vi "Acquire Data.vi"(8 "error in (no error)":errorcluster, 11 "USB Camera in":refnum<class "USB Camera.lvclass">) -> (0 "error out":errorcluster, 3 "USB Camera out":refnum<class "USB Camera.lvclass">)   [LabVIEW 2020, in "USB Camera.lvclass"]
uses:
  USB Camera.lvclass
  C:/Users/jharw/Documents/1 Folder to Rule them All/UMD/Inflation-Apparatus/src/Hardware/Sensors/Cameras/Camera.lvclass
  C:/Users/jharw/Documents/1 Folder to Rule them All/UMD/Inflation-Apparatus/src/Hardware/General Hardware.lvclass
  <vilib>/vision/driver/IMAQdx.llb/IMAQdx Buffer Number Mode.ctl
  General Hardware.lvclass/General Hardware.ctl
  USB Camera.lvclass/USB Camera.ctl
  Camera.lvclass/Camera.ctl
  Camera.lvclass
  General Hardware.lvclass
  <vilib>/vision/driver/NI_Vision_Acquisition_Software.lvlib
  <vilib>/vision/NI_Vision_Development_Module.lvlib
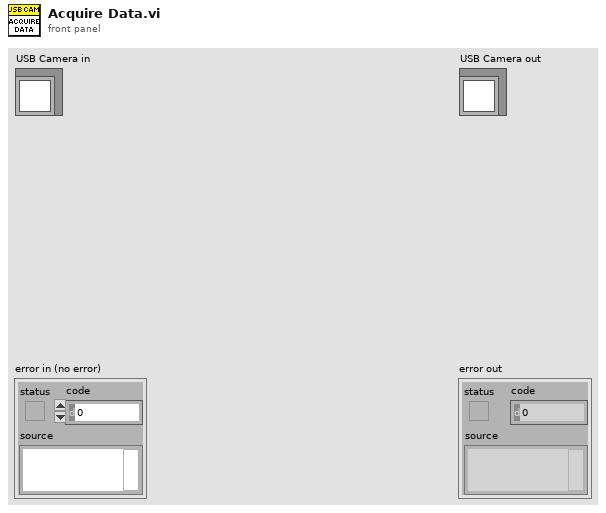
[diagram p1: front panel]
types:
  T1 = cluster{"Contrast":i32, "Filter width":i32, "Steepness":i32, "Subsampling Ratio":u32, "Show Search Area":bool, "Show Search Lines":bool, "Show Edges Found":bool, "Show Result":bool}
  T2 = typedef "NI_Vision_Acquisition_Software.lvlib/IMAQdx Buffer Number Mode.ctl" = enum32{"Next", "Last", "Buffer Number", "Every", "Last New"}
  T3 = typedef "IMAQdx.ctl" = refnum<k21>
  T4 = typedef "IMAQ Image.ctl" = refnum<image>
  T5 = typedef "IMAQ Rectangle" = cluster{"Left":i32, "Top":i32, "Right":i32, "Bottom":i32, "Rotation":dbl}
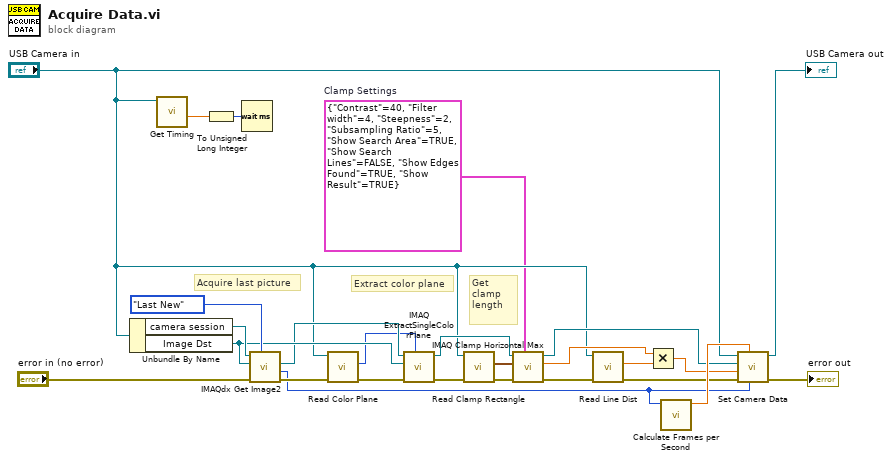
[diagram p0: block diagram]
diagram:
  w3 = T1 {"Contrast"=40, "Filter width"=4, "Steepness"=2, "Subsampling Ratio"=5, "Show Search Area"=TRUE, "Show Search Lines"=FALSE, "Show Edges Found"=TRUE, "Show Result"=TRUE}  # Clamp Settings
  # "Get clamp length"
  # "Extract color plane"
  # "Acquire last picture"
  n1 = Unbundle By Name("USB Camera in") -> ("camera session"=w20:T3, "Image Dst"=w16:T4)
  n2 = call "Get Timing.vi"("General Hardware in"="USB Camera in") -> ("time delay (ms)"=w22:dbl)  [unwired: 7 in, 3 out]
  n3 = To Unsigned Long Integer(number=w22) -> (unsigned 32bit integer=w23:u32)
  n4 = Wait (ms)(milliseconds to wait=w23) -> ()  [unwired: 1 out]
  n5 = call <vilib>:"IMAQdx Get Image2.vi"("Buffer Number Mode (Next)"=IMAQdx_Buffer_Number_Mode."Last New" ("Buffer Number Mode"), "error in"="error in (no error)", "Image In"=w16, "Session In"=w20) -> ("error out"=w18:errorcluster, "Buffer Number Out"=w2:u32, "Image Out"=w15:T4)  [unwired: 4 in, 1 out]
  n6 = call "Read Color Plane.vi"("error in (no error)"=w18, "Camera in"="USB Camera in") -> ("error out"=w17:errorcluster, "Color Plane"=w1:i32)  [unwired: 7 in, 1 out]
  n7 = call "IMAQ ExtractSingleColorPlane"("Color Plane"=w1, "error in (no error)"=w17, "Image Dst"=w16, "Image Src"=w15) -> ("error out"=w14:errorcluster, "Image Dst Out"=w11:T4)  [unwired: 6 in]
  n8 = call "Read Clamp Rectangle.vi"("error in (no error)"=w14, "Camera in"="USB Camera in") -> ("error out"=w13:errorcluster, "Rectangle"=w12:T5)  [unwired: 7 in, 1 out]
  n9 = call "IMAQ Clamp Horizontal Max"("Settings"=w3, "error in (no error)"=w13, "Rectangle"=w12, "Image"=w11) -> ("error out"=w9:errorcluster, "Distance"=w7:sgl, "Image Out"=w10:T4)  [unwired: 3 in, 2 out]
  n10 = call "Read Line Dist.vi"("error in (no error)"=w9, "Camera in"="USB Camera in") -> ("error out"=w4:errorcluster, "mm/pixel"=w8:dbl)  [unwired: 7 in, 1 out]
  n11 = Multiply(x=w7, y=w8) -> (x*y=w5:dbl)
  n12 = call <vilib>:"Calculate Frames per Second.vi"("Buffer Number"=w2) -> ("Acquired Frames/s"=w25:dbl)  [unwired: 8 in, 2 out]
  n13 = call "Set Camera Data.vi"("cam buffer"=w2, "cam framerate"=w25, "error in (no error)"=w4, "diameter (mm)"=w5, "image"=w10, "Camera in"="USB Camera in") -> ("error out"=→"error out":errorcluster, "Camera out"=→"USB Camera out":refnum<class "USB Camera.lvclass">)  [unwired: 4 in]
